vi "Daemon.vi"(8 "error in (no error)":errorcluster, 10 "Return Queue":refnum<queue>, 11 "MenuButton Event Handler in":refnum<class "MenuButton Event Handler.lvclass">) -> ()   [LabVIEW 2017, in "MenuButtons.lvlib" / "MenuButton Event Handler.lvclass"]
uses:
  MenuButton Event Handler.lvclass
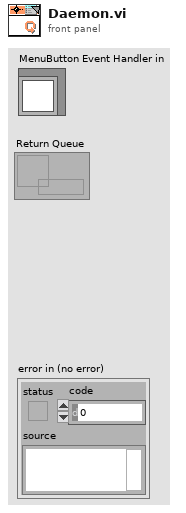
[diagram p1: front panel]
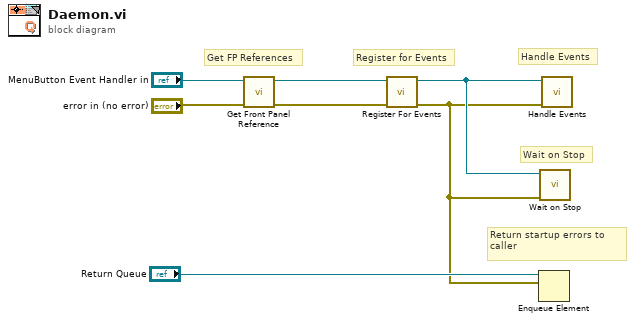
[diagram p0: block diagram]
diagram:
  # "Return startup errors to caller"
  # "Wait on Stop"
  # "Handle Events"
  # "Register for Events"
  # "Get FP References"
  n1 = call "Get Front Panel Reference.vi"("error in (no error)"="error in (no error)", "MenuButton Event Handler in"="MenuButton Event Handler in") -> ("error out"=w4:errorcluster, "MenuButton Event Handler out"=w5:refnum<class "MenuButton Event Handler.lvclass">)  [unwired: 8 in]
  n2 = call "Register For Events.vi"("error in (no error)"=w4, "MenuButton Event Handler in"=w5) -> ("error out"=w1:errorcluster, "MenuButton Event Handler out"=w7:refnum<class "MenuButton Event Handler.lvclass">)  [unwired: 8 in]
  n3 = Enqueue Element(queue="Return Queue", element=w1) -> ()  [unwired: 2 in, 3 out]
  n4 = call "Wait on Stop.vi"("error in (no error)"=w1, "MenuButton Event Handler in"=w7) -> ()  [unwired: 10 in]
  n5 = call "Handle Events.vi"("error in (no error)"=w1, "MenuButton Event Handler in"=w7) -> ()  [unwired: 10 in]
